vi "Tri-State High Impedance.vi"(8 "error in":errorcluster, 11 "output terminal":tag) -> (0 "error out":errorcluster)   [LabVIEW 2018]
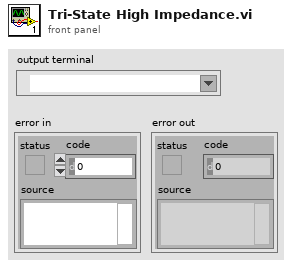
[diagram p1: front panel]
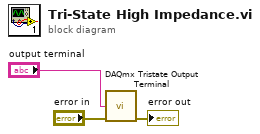
[diagram p0: block diagram]
diagram:
  n1 = call <vilib>:"DAQmx Tristate Output Terminal.vi"("output terminal"="output terminal", "error in"="error in") -> ("error out"=→"error out":errorcluster)  [unwired: 13 in]
